vi "A 侧面 处理函数衬丝检测.vi"(8 "error in (no error)":errorcluster caption="错误输入（无错误）", 9 "Session in":T1, 10 "Image Name":string="I1", 11 "CR-检测基础参数":T2={"IsNorImage"=TRUE, "Exposure Values"=100289, "ImagePath"=path "C:/Users/hedongpo/Desktop/514-hdp/Alignment Assemble System/Test Picture/B/3.bmp"} caption="参数界面" {"Exposure Values" scale=0.0..200000.0}) -> (0 "error out":errorcluster caption="错误输出", 2 "Session Out":T1, 3 "Image out":T3(plugin-control), 4 "数值":dbl)   [LabVIEW 2017]
uses:
  <vilib>/userdefined/High Color/IMAQdx.ctl
  <vilib>/vision/driver/IMAQdx.llb/IMAQdx Buffer Number Mode.ctl
  <resource>/objmgr/imaqdx.rc
  Global System.vi
  <vilib>/vision/driver/NI_Vision_Acquisition_Software.lvlib
  <vilib>/vision/NI_Vision_Development_Module.lvlib
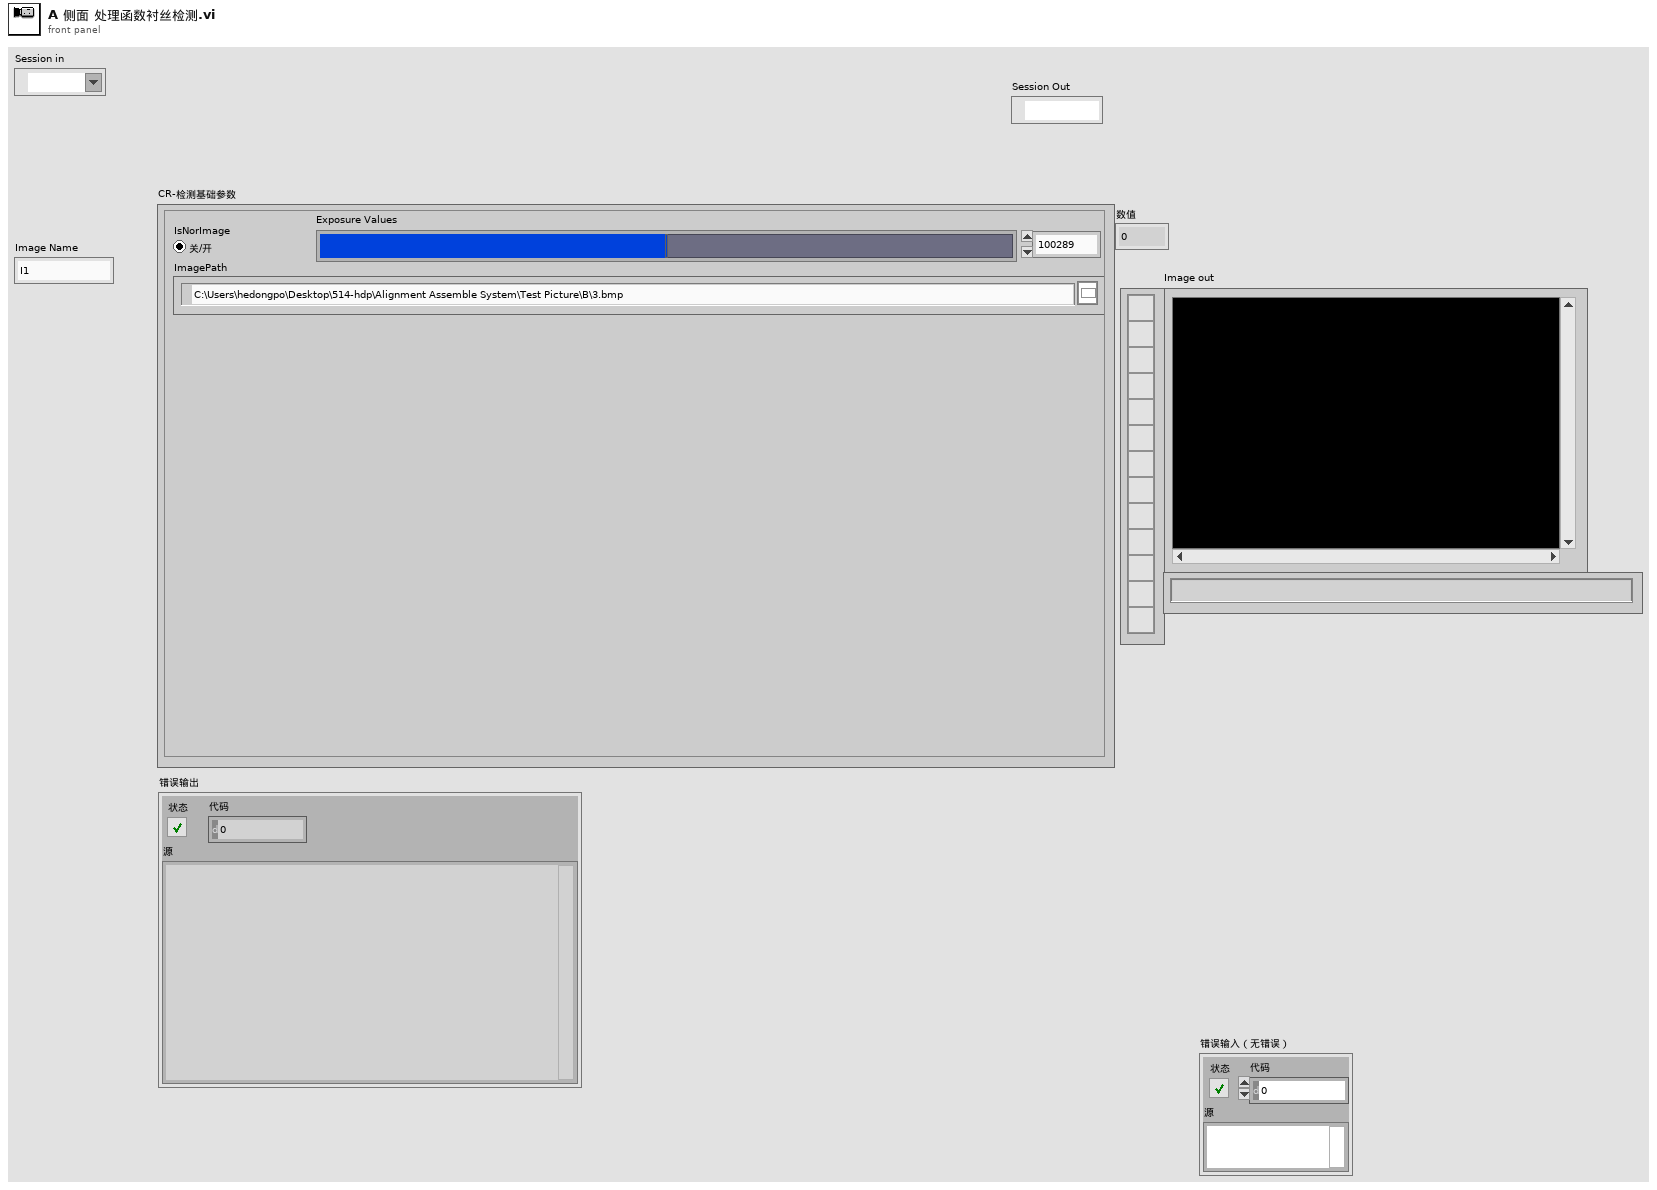
[diagram p1: front panel]
types:
  T1 = typedef "IMAQdx.ctl" = refnum<k21>
  T2 = cluster{"IsNorImage":bool, "Exposure Values":i64, "ImagePath":path}
  T3 = typedef "IMAQ Image.ctl" = refnum<image>
  T4 = typedef "Image Type" = u32
  T5 = cluster{"IsNorImage":bool, "Exposure Values":u32, "ImagePath":path}
  T6 = typedef "NI_Vision_Acquisition_Software.lvlib/IMAQdx Buffer Number Mode.ctl" = enum32{"Next", "Last", "Buffer Number", "Every", "Last New"}
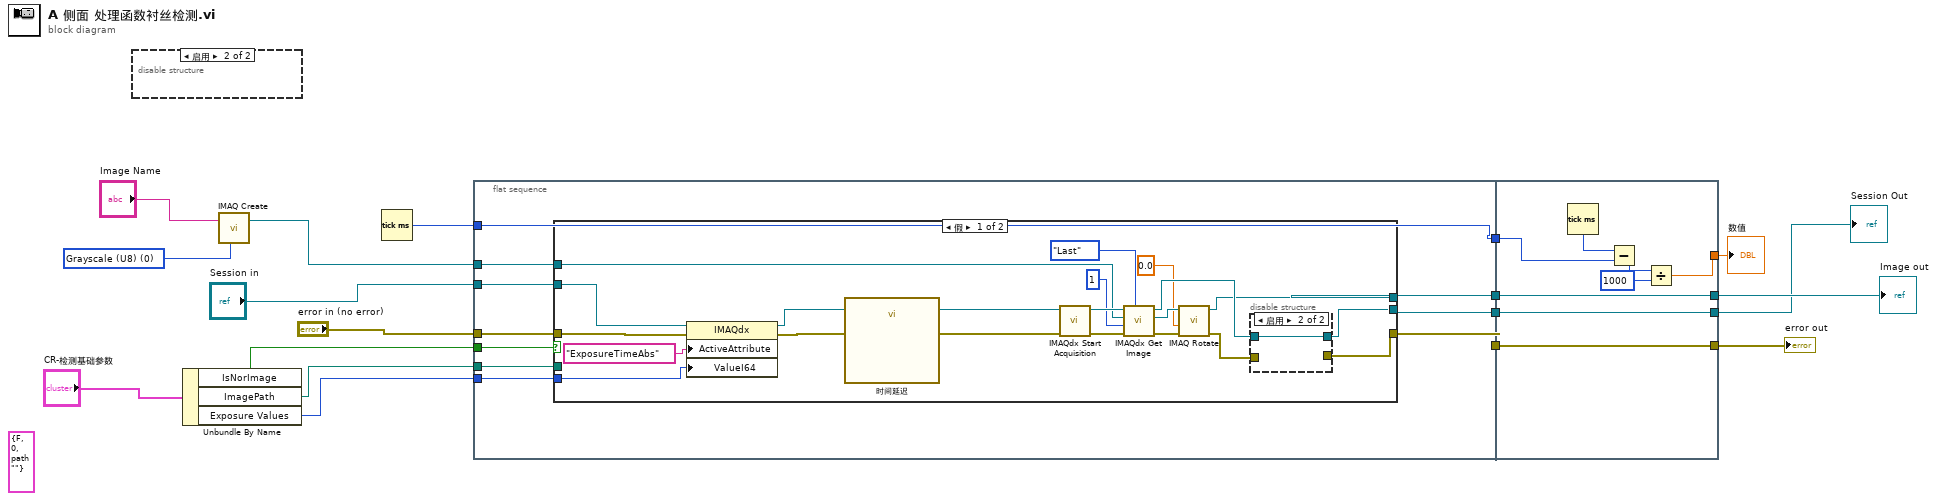
[diagram p0: block diagram]
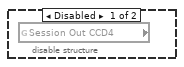
[diagram p2: hidden frame]
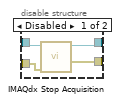
[diagram p3: hidden frame]
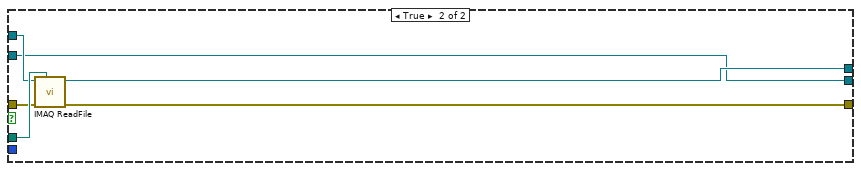
[diagram p4: hidden frame]
diagram:
  w13 = T4 0 items=["Grayscale (U8)", "Grayscale (I16)", "Grayscale (SGL)", "Complex (CSG)", "RGB (U32)", "HSL (U32)", "RGB (U64)", "Grayscale (U16)"] ("Image Type")
  (unwired) T5 {"IsNorImage"=FALSE, "Exposure Values"=0, "ImagePath"=path ""} ("ParamsUI")
  n1 = disable-structure shown="启用" {
    frame Disabled {
      n2 = global read "Global System.vi" "Session Out CCD4"() -> ()  [unwired: 1 out]
    }
    frame Enabled {
    }
  }
  n3 = Unbundle By Name("CR-检测基础参数") -> ("IsNorImage"=w2:bool, "ImagePath"=w3:path, "Exposure Values"=w18:i64)
  n4 = call "IMAQ Create"("Image Name"="Image Name", "Image Type"=w13) -> ("New Image"=w16:T3)  [unwired: 3 in, 1 out]
  n5 = Tick Count (ms)() -> (millisecond timer value=w9:u32)
  n6 = flat-sequence {
    tunnel: w2 -> [w28]
    tunnel: w3 -> [w27]
    tunnel: w18 -> [w26]
    tunnel: w16 -> [w25]
    tunnel: "error in (no error)" -> [w24]
    tunnel: "Session in" -> [w21]
    tunnel: w9 -> [w19]
    tunnel: [w23] -> w8
    tunnel: [w22] -> w7
    tunnel: [w20] -> w6
    tunnel: [w19] -> w5
    tunnel: [w65] -> w10
    tunnel: [w66] -> w11
    tunnel: [w67] -> w14
    tunnel: w8 -> [w67]
    tunnel: w7 -> [w66]
    tunnel: w6 -> [w65]
    tunnel: w5 -> [w63]
    tunnel: [w60] -> w4
    frame #0 {
      n7 = case shown="假" w28 {
        tunnel: w27 -> [_ w59]
        tunnel: [w38 w58] -> w22
        tunnel: w26 -> [w33 _]
        tunnel: w21 -> [w35 w54]
        tunnel: w25 -> [w39 w57]
        tunnel: w24 -> [w34 w56]
        tunnel: [w36 w55] -> w23
        tunnel: [w37 w54] -> w20
        frame False {
          n8 = property class="IMAQdx"(reference=w35, error in=w34, "ActiveAttribute"="ExposureTimeAbs", "ValueI64"=w33) -> (reference out=w32:T1, error out=w31:errorcluster)
          n9 = call "时间延迟"("error in (no error)"=w31) -> ("error out"=w29:errorcluster)  [unwired: 10 in]
          n10 = call <vilib>:"IMAQdx Start Acquisition.vi"("error in"=w29, "Session In"=w32) -> ("error out"=w47:errorcluster, "Session Out"=w48:T1)  [unwired: 8 in]
          n11 = call <vilib>:"IMAQdx Get Image.vi"("Buffer Number Mode (Next)"=IMAQdx_Buffer_Number_Mode."Last", "error in"=w47, "Buffer Number In"=u32 1, "Image In"=w39, "Session In"=w48) -> ("error out"=w42:errorcluster, "Image Out"=w43:T3, "Session Out"=w44:T1)  [unwired: 3 in, 1 out]
          n12 = call "IMAQ Rotate"("error in (no error)"=w42, "Angle (degrees)"=sgl 0.0, "Image Src"=w43) -> ("error out"=w41:errorcluster, "Image Dst Out"=w38:T3)  [unwired: 7 in]
          n13 = disable-structure shown="启用" {
            disable-tunnel: w44 -> [w52 w53]
            disable-tunnel: w41 -> [w51 _]
            disable-tunnel: [w50 w53] -> w37
            disable-tunnel: [w49 _] -> w36
            frame Disabled {
              n14 = call <vilib>:"IMAQdx Stop Acquisition.vi"("error in"=w51, "Session In"=w52) -> ("error out"=w49:errorcluster, "Session Out"=w50:T1)  [unwired: 8 in]
            }
            frame Enabled {
            }
          }
        }
        frame True {
          n15 = call "IMAQ ReadFile"("File Path"=w59, "error in (no error)"=w56, "Image"=w57) -> ("error out"=w55:errorcluster, "Image Out"=w58:T3)  [unwired: 4 in, 3 out]
        }
      }
    }
    frame #1 {
      n16 = Tick Count (ms)() -> (millisecond timer value=w64:u32)
      n17 = Subtract(x=w64, y=w63) -> (x-y=w62:u32)
      n18 = Divide(x=w62, y=u32 1000) -> (x/y=w60:dbl)
    }
  }
  "Image out" <- w11
  "error out" <- w14
  "Session Out" <- w10
  "数值" <- w4
